vi "GetStartStopCommand.vi"(11 "Run Chamber":bool=TRUE) -> (3 "Command":u8[](array[numeric]) format="%x")   [LabVIEW 2015]
uses:
  <instrlib>/Samwontech TEMP2xxx/Samwontech TEMP2xxx.lvlib
panel:
  out "Command":string
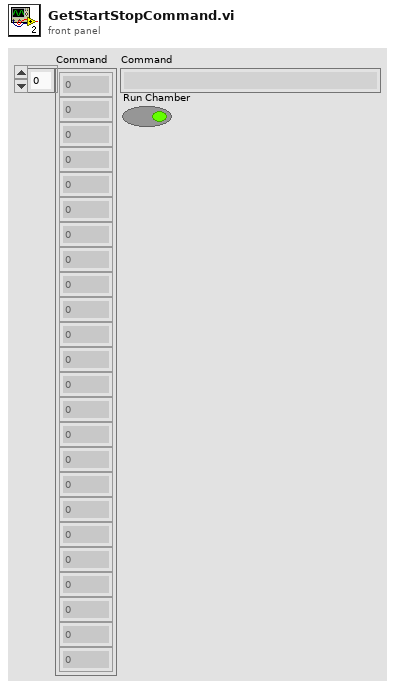
[diagram p1: front panel]
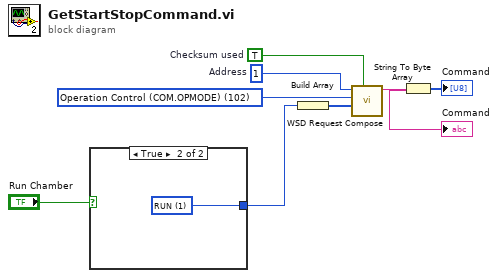
[diagram p0: block diagram]
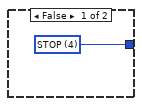
[diagram p2: hidden frame]
diagram:
  w7 = u8 1  # Address
  w8 = TRUE  # Checksum used
  w6 = u32 102 items=["Current PV (NPV)"=1, "Operation Control (COM.OPMODE)"=102, "Set Point on FIX operation (FIX.TSP)"=104, "Operation Mode (OP.MODE)"=106] ("D-Registers Map")
  n1 = case shown="True" "Run Chamber" {
    tunnel: [w9 w10] -> w1
    frame False {
      w9 = u32 4 items=["RUN"=1, "HOLD"=2, "STEP"=3, "STOP"=4] ("Mode Control")
    }
    frame True {
      w10 = u32 1 items=["RUN"=1, "HOLD"=2, "STEP"=3, "STOP"=4] ("Mode Control")
    }
  }
  n2 = Build Array(w1) -> (w5:u32[])
  n3 = call <instrlib>:"WSD Request Compose.vi"("Checksum used"=w8, "Data"=w5, "D-register number"=w6, "Address"=w7) -> ("Request"=w4:string)  [unwired: 6 in, 1 out]
  "Command" <- w4
  n4 = String To Byte Array(string=w4) -> (unsigned byte array=→"Command":u8[])
